vi "Terminal_Work_Condition.vi"   [LabVIEW 2014]
uses:
  Work_Condition.vi
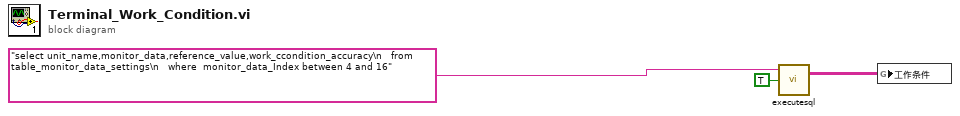
[diagram p0: block diagram]
diagram:
  n1 = call "executesql.vi"("Return Data (T)"=TRUE, "Command Text"="select unit_name,monitor_data,reference_value,work_ccondition_accuracy\n   from table_monitor_data_settings\n   where  monitor_data_Index between 4 and 16") -> ("Data"=w1:string[][])  [unwired: 5 in, 1 out]
  n2 = global write "Work_Condition.vi" "工作条件"(w1) -> ()
